vi "UTiLIA Main.vi"() -> ()   [LabVIEW 2022 SP3]
uses:
  <vilib>/Analysis/NI_AALPro.lvlib
  <vilib>/Analysis/5stat.llb/RMS (DBL).vi
  <vilib>/Utility/file.llb/Write To Spreadsheet File (DBL).vi
panel:
  in  "Sim?":bool
  out "Avg Temperature":dbl=296.9343435186893 format="%.1f"
  out "Nominal Resistance":dbl=0.0029999351419545705 format="%.2e"
  in  "Nom. Amplification":u16(ring)=3 items=["1", "10", "100", "1000", "10000"]
  out "Avg Quadrature Volt":dbl=-9.334672475592858e-06 format="%.5f"
  out "Long Avg Samp Volt":dbl=0.7499993324589096 format="%.6f"
  out "Avg Samp Volt":dbl=0.7499837854886428 format="%.6f"
  out "Measured Current":dbl=0.25000000000000006 format="%.0p"
  in  "Desired Current":dbl=0.25 format="%.0p"
  in  "Stop!":bool
  out "N=":i32=53
  in  "Calculate FFT?":bool=TRUE
  in  "Reset Avg?":bool
  out "Sampling Info":cluster{dbl[unit], i32}={71808.0, 16384} {"Hz" format="%.2f"}
  out "#S":i32=16384 caption="Samp/Chk"
  out "s/Samp":dbl[unit]=1.392602495543672e-05 format="%.0p"
  out "Fs":dbl[unit]=71808.0 caption="Samp Freq"
  out "Backlog":u32
  out "s/Chunk":dbl[unit]=0.2281639928698752 format="%.2f"
  out "s/Iter":dbl[unit]=0.13100000000849832 format="%.0p"
  in  "Reset Graph?":bool
  out "Resistance vs. Temp":cluster{dbl, dbl}[](graph)
  out "Error out":errorcluster
  in  "Save?":bool
  in  "Append?":bool
  in  "Data File":path=path "c:/users/flip/data/Test.txt"
  in  "Scale SV":dbl=1.0 min=0.0 max=2000.0 step=1.0 format="%.1p"
  out "Waveforms":dbl[][](graph)
  out "Mult Q":dbl[](array[numeric]) format="%.2f"
  out "Unit Reference":dbl[](array[numeric]) format="%.2f"
  out "Mult IP":dbl[](array[numeric]) format="%.2f"
  out "Applied Current":dbl[](array[numeric]) format="%.2f"
  out "Sample Voltage":dbl[](array[numeric]) format="%.2f"
  in  "Ref Freq":dbl[unit]=1122.0
  in  "Fs/Fref":u16=64 max=2000 step=20
  in  "Log S":i8=14 min=0 max=20 step=1
  out "Settle Time":dbl[unit]=0.025 format="%.1p"
  in  "Cutoff Freq":dbl[unit]=40.0 format="%.1f"
  in  "Filter Type":T1(ring)=enum."Inv Chebyshev"
  out "Avg Voltage vs. Time":T2(graph)={"Chunk Average"=0.7499837854886428, "Long-term Average"=0.7499993324589096, "Chunk Average"=-9.334672475592858e-06, 0.29693434351868925}
  out "FFT of Signal":cluster{"x":dbl, "df":dbl, dbl[]}[](graph)=[{"x"=0.0, "df"=4.3828125, array[8192 elements]}, {"x"=0.0, "df"=4.3828125, array[8192 elements]}, {"x"=0.0, "df"=4.3828125, array[8192 elements]}]
  out "Uncertainty Estimate":dbl[](graph)=[1.5546970266844262e-05]
  # "Save Data to File"
  # "Sampling Info"
  # "Averaged Values"
  # "Filter Info"
  # "Error Status"
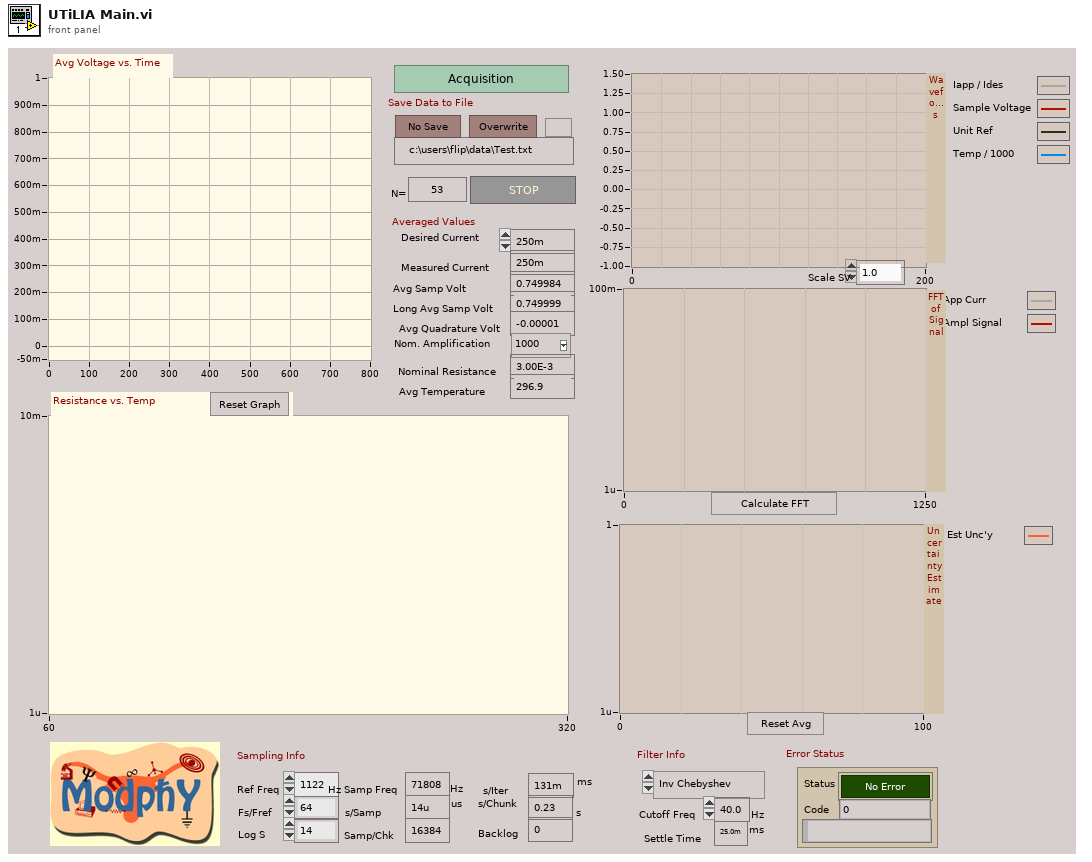
[diagram p1: front panel]
types:
  T1 = enum16{"None", "Butterworth", "Chebyshev", "Inv Chebyshev"}
  T2 = cluster{"Chunk Average":dbl, "Long-term Average":dbl, "Chunk Average":dbl, dbl}
  T3 = cluster{"Average mode":enum16{"No Averaging", "Linear", "Exponential"}, "# of averages":u32}
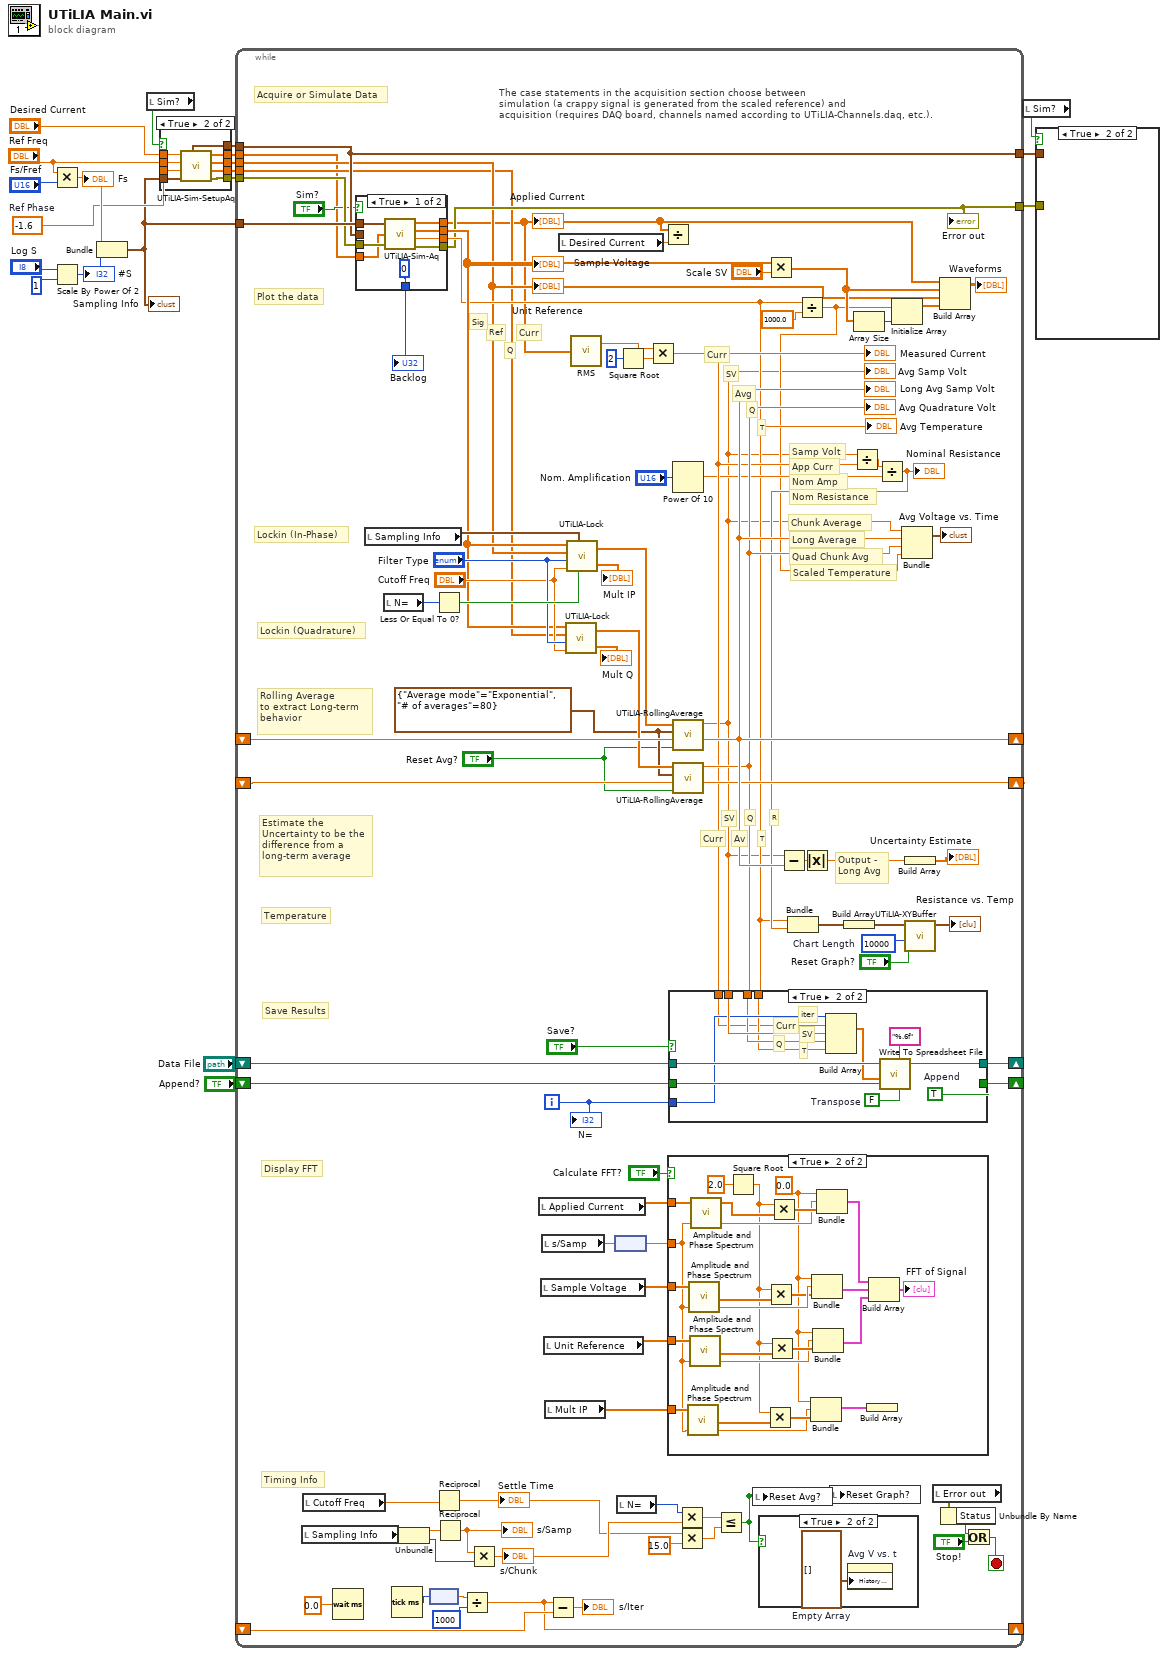
[diagram p0: block diagram]
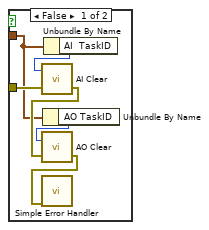
[diagram p2: hidden frame]
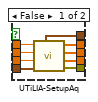
[diagram p3: hidden frame]
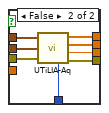
[diagram p4: hidden frame]
diagram:
  w6 = -1.6  # Ref Phase
  n1 = Multiply(x="Ref Freq", y="Fs/Fref") -> (x*y=w11:dbl[unit])
  "Fs" <- w11
  n2 = Scale By Power Of 2(n="Log S", x=1 ("n")) -> (x*2^n=w10:i32)
  "#S" <- w10
  n3 = Bundle(w11, w10) -> (w5:cluster{dbl[unit], i32})  [unwired: 1 in]
  "Sampling Info" <- w5
  n4 = local read "Sim?"() -> (w3:bool)
  n5 = case shown="True" w3 {
    tunnel: [w29 w38] -> w18
    tunnel: [w28 w37] -> w4
    tunnel: [w27 w36] -> w16
    tunnel: [w26 w35] -> w15
    tunnel: "Ref Freq" -> [w25 w34]
    tunnel: w5 -> [w24 w33]
    tunnel: "Desired Current" -> [w23 w32]
    tunnel: w6 -> [w22 w31]
    tunnel: [w21 w30] -> w2
    frame False {
      n6 = call "UTiLIA-SetupAq.vi"("Sampling Info"=w24, "Ref Phase"=w22, "Ref Frequency"=w25, "Ref Amplitude"=w23) -> ("Error out"=w29:errorcluster, "Unit Quadrature"=w26:dbl[], "Unit Reference"=w27:dbl[], "Scaled Reference"=w21:dbl[], "DAQ Configuration"=w28:cluster{"AO TaskID":u32, "AI  TaskID":u32})
    }
    frame True {
      n7 = call "UTiLIA-Sim-SetupAq.vi"("Sampling Info"=w33, "Ref Phase"=w31, "Ref Frequency"=w34, "Ref Amplitude"=w32) -> ("Error out"=w38:errorcluster, "Unit Quadrature"=w35:dbl[], "Unit Reference"=w36:dbl[], "Scaled Reference"=w30:dbl[], "DAQ Configuration"=w37:cluster{"AO TaskID":u32, "AI  TaskID":u32})
    }
  }
  n8 = while {
    shift-right: [w128] -> _
    shift-left: "Data File" -> [w127]
    shift-right: [w121] -> _
    shift-left: "Append?" -> [w126]
    shift-right: [w96] -> _
    shift-left: _ -> [w116]
    tunnel: w5 -> [w106]
    tunnel: w18 -> [w105]
    tunnel: [w55] -> w17
    tunnel: [w102] -> w9
    tunnel: w4 -> [w102]
    tunnel: w16 -> [w43]
    tunnel: w15 -> [w42]
    shift-right: [w59] -> _
    shift-left: _ -> [w87]
    shift-right: [w75] -> _
    shift-left: _ -> [w76]
    tunnel: w2 -> [w40]
    i -> [w107]
    stop <- w82 stop-if-true
    w74 = 10000  # Chart Length
    w77 = T3 {"Average mode"=enum."Exponential", "# of averages"=80} ("Rolling Avg Params")
    # "Plot the data"
    # "Acquire or Simulate Data"
    # "The case statements in the acquisition section choose between \nsimulation (a crappy signal is generated from the scaled reference) and\nacquisition (requires DAQ board, channels named according to UTiLIA-Channels.daq, etc.)."
    # "Curr"
    # "Nom Amp"
    # "Scaled Temperature"
    # "R"
    # "Nom Resistance"
    # "App Curr"
    # "Samp Volt"
    # "Quad Chunk Avg"
    # "Av"
    # "Curr"
    # "Curr"
    # "Q"
    # "Timing Info"
    # "Avg"
    # "T"
    # "SV"
    # "Q"
    # "Q"
    # "SV"
    # "Temperature"
    # "Display FFT"
    # "Save Results"
    # "T"
    # "Ref"
    # "Sig"
    # "Estimate the\nUncertainty to be the\ndifference from a \nlong-term average"
    # "Output -\nLong Avg"
    # "Long Average"
    # "Chunk Average"
    # "Rolling Average\nto extract Long-term \nbehavior"
    # "Lockin (Quadrature)"
    # "Lockin (In-Phase)"
    n9 = local read "Sampling Info"() -> (w125:cluster{dbl[unit], i32})
    n10 = local read "Cutoff Freq"() -> (w120:dbl[unit])
    n11 = Wait (ms)(milliseconds to wait=0.0) -> ()  [unwired: 1 out]
    n12 = case shown="True" "Sim?" {
      tunnel: w106 -> [w131 w144]
      tunnel: w105 -> [w136 w143]
      tunnel: [u32 0 ("Backlog") w142] -> w104
      tunnel: w102 -> [_ w141]
      tunnel: [w135 w140] -> w80
      tunnel: [w134 w139] -> w39
      tunnel: [w132 w138] -> w61
      tunnel: [w133 w137] -> w55
      tunnel: w40 -> [w130 _]
      frame True {
        n13 = call "UTiLIA-Sim-Aq.vi"("Sampling Info"=w131, "Scaled Reference"=w130, "Error in"=w136) -> ("Applied Current"=w134:dbl[], "Sample Voltage"=w135:dbl[], "Avg Temperature"=w132:dbl, "Error out"=w133:errorcluster)  [unwired: 1 in]
      }
      frame False {
        n14 = call "UTiLIA-Aq.vi"("Sampling Info"=w144, "DAQ Configuration"=w141, "Error in"=w143) -> ("Applied Current"=w139:dbl[], "Sample Voltage"=w140:dbl[], "Avg Temperature"=w138:dbl, "Error out"=w137:errorcluster, "Backlog"=w142:u32)
      }
    }
    "Backlog" <- w104
    "Sample Voltage" <- w80
    "Applied Current" <- w39
    "Avg Temperature" <- w61
    "Error out" <- w55
    n15 = local read "Sampling Info"() -> (w99:cluster{dbl[unit], i32})
    n16 = local read "N="() -> (w114:i32)
    n17 = Tick Count (ms)() -> (millisecond timer value=w88:u32)
    n18 = Unbundle(w125) -> (w123:dbl[unit], w124:i32)
    n19 = node(w88) -> (w54:dbl[unit])
    n20 = Less Or Equal To 0?(x=w114) -> (x <= 0?=w100:bool)
    n21 = Reciprocal(x=w120) -> (1/x=w110:dbl[unit])
    "Settle Time" <- w110
    n22 = Reciprocal(x=w123) -> (1/x=w122:dbl[unit])
    "s/Samp" <- w122
    n23 = Divide(x=w54, y=u32 1000) -> (x/y=w59:dbl[unit])
    n24 = Multiply(x=w122, y=w124) -> (x*y=w112:dbl[unit])
    "s/Chunk" <- w112
    n25 = local read "Applied Current"() -> (w90:dbl[])
    n26 = local read "Sample Voltage"() -> (w89:dbl[])
    n27 = local read "s/Samp"() -> (w49:dbl[unit])
    n28 = local read "Unit Reference"() -> (w91:dbl[])
    n29 = local read "Mult IP"() -> (w115:dbl[])
    n30 = Subtract(x=w59, y=w87) -> (x-y=→"s/Iter":dbl[unit])
    n31 = local read "Desired Current"() -> (w44:dbl)
    n32 = call "UTiLIA-Lock.vi"("Cutoff Freq"="Cutoff Freq", "Filter Type"="Filter Type", "Unit Reference"=w42, "Noisy Signal"=w80) -> ("Multiplied Signal"=→"Mult Q":dbl[], "Locked Signal"=w78:dbl[])  [unwired: 2 in]
    n33 = call "UTiLIA-Lock.vi"("Reset Filter?"=w100, "Sampling Info"=w99, "Cutoff Freq"="Cutoff Freq", "Filter Type"="Filter Type", "Unit Reference"=w43, "Noisy Signal"=w80) -> ("Multiplied Signal"=→"Mult IP":dbl[], "Locked Signal"=w97:dbl[])
    n34 = call-poly <vilib>:"RMS.vi"("X"=w39) -> ("rms value"=w67:dbl)  [unwired: 1 out]
    n35 = node(w49) -> (w50:dbl)
    n36 = local read "N="() -> (w113:i32)
    n37 = Square Root(x=2 ("y")) -> (sqrt(x)=w68:dbl)
    n38 = Multiply(x=w67, y=w68) -> (x*y=w66:dbl)
    "Measured Current" <- w66
    n39 = Divide(x=w39, y=w44) -> ()  [unwired: 1 out]
    n40 = case shown="True" "Calculate FFT?" {
      tunnel: w90 -> [_ w168]
      tunnel: w115 -> [_ w163]
      tunnel: w50 -> [_ w146]
      tunnel: w89 -> [_ w154]
      tunnel: w91 -> [_ w153]
      frame False {
      }
      frame True {
        w149 = 0.0 ("x")
        n41 = call <vilib>:"Amplitude and Phase Spectrum.vi"("dt"=w146, "Signal (V)"=w163) -> ("df"=w161:dbl, "Amp Spectrum Mag (Vrms)"=w164:dbl[])  [unwired: 1 in, 1 out]
        n42 = call <vilib>:"Amplitude and Phase Spectrum.vi"("dt"=w146, "Signal (V)"=w154) -> ("df"=w160:dbl, "Amp Spectrum Mag (Vrms)"=w159:dbl[])  [unwired: 1 in, 1 out]
        n43 = call <vilib>:"Amplitude and Phase Spectrum.vi"("dt"=w146, "Signal (V)"=w153) -> ("df"=w150:dbl, "Amp Spectrum Mag (Vrms)"=w151:dbl[])  [unwired: 1 in, 1 out]
        n44 = call <vilib>:"Amplitude and Phase Spectrum.vi"("dt"=w146, "Signal (V)"=w168) -> ("df"=w166:dbl, "Amp Spectrum Mag (Vrms)"=w169:dbl[])  [unwired: 1 in, 1 out]
        n45 = Square Root(x=2.0) -> (sqrt(x)=w148:dbl)
        n46 = Multiply(x=w148, y=w164) -> (x*y=w165:dbl[])
        n47 = Multiply(x=w148, y=w159) -> (x*y=w158:dbl[])
        n48 = Multiply(x=w148, y=w151) -> (x*y=w152:dbl[])
        n49 = Multiply(x=w148, y=w169) -> (x*y=w167:dbl[])
        n50 = Bundle("x"=w149, "df"=w161, w165) -> (w162:cluster{"x":dbl, "df":dbl, dbl[]})  [unwired: 1 in]
        n51 = Bundle("x"=w149, "df"=w160, w158) -> (w155:cluster{"x":dbl, "df":dbl, dbl[]})  [unwired: 1 in]
        n52 = Bundle("x"=w149, "df"=w150, w152) -> (w147:cluster{"x":dbl, "df":dbl, dbl[]})  [unwired: 1 in]
        n53 = Bundle("x"=w149, "df"=w166, w167) -> (w156:cluster{"x":dbl, "df":dbl, dbl[]})  [unwired: 1 in]
        n54 = Build Array(w162) -> ()  [unwired: 1 out]
        n55 = Build Array(w156, w155, w147) -> (→"FFT of Signal":cluster{"x":dbl, "df":dbl, dbl[]}[])
      }
    }
    n56 = Power Of 10(x="Nom. Amplification") -> (10^x=w63:dbl)
    n57 = call "UTiLIA-RollingAverage.vi"("Restart Avg"="Reset Avg?", "Current Average"=w116, "Rolling Avg Parameters"=w77, "Signal to Average"=w97) -> ("Long-term Average"=w96:dbl, "Chunk Average"=w48:dbl)  [unwired: 3 out]
    "Avg Samp Volt" <- w48
    "Long Avg Samp Volt" <- w96
    n58 = call "UTiLIA-RollingAverage.vi"("Restart Avg"="Reset Avg?", "Current Average"=w76, "Rolling Avg Parameters"=w77, "Signal to Average"=w78) -> ("Long-term Average"=w75:dbl, "Chunk Average"=w71:dbl)  [unwired: 3 out]
    "Avg Quadrature Volt" <- w71
    n59 = case shown="True" "Save?" {
      tunnel: [w172 w183] -> w128
      tunnel: w127 -> [w172 w182]
      tunnel: w126 -> [w171 w181]
      tunnel: [w171 w179] -> w121
      tunnel: w48 -> [_ w178]
      tunnel: w61 -> [_ w174]
      tunnel: w107 -> [_ w176]
      tunnel: w71 -> [_ w175]
      tunnel: w66 -> [_ w173]
      frame False {
      }
      frame True {
        w179 = TRUE  # Append
        w180 = FALSE  # Transpose
        # "Curr"
        # "Q"
        # "SV"
        # "T"
        # "iter"
        n60 = Build Array(w176, w173, w178, w175, w174) -> (w177:dbl[])
        n61 = call-poly <vilib>:"Write To Spreadsheet File.vi"("transpose? (no:F)"=w180, "format (%.3f)"="%.6f", "append to file? (new file:F)"=w181, "1D data"=w177, "file path (dialog if empty)"=w182) -> ("new file path (Not A Path if cancelled)"=w183:path)  [unwired: 3 in]
      }
    }
    n62 = Multiply(x=w113, y=w112) -> (x*y=w111:dbl[unit])
    n63 = Multiply(x=w110, y=15.0 ("x")) -> (x*y=w109:dbl[unit])
    n64 = Less Or Equal?(x=w111, y=w109) -> (x <= y?=w45:bool)
    n65 = local write "Reset Avg?"(w45) -> ()
    n66 = case shown="True" w45 {
      frame False {
      }
      frame True {
        w145 = cluster{dbl, dbl, dbl, dbl}[] []  # Empty Array
        n67 = property on="Avg V vs. t" class="WFChart (strict)"("History Data"=w145) -> ()  [unwired: 2 in, 2 out]
      }
    }
    n68 = Multiply(x=w80, y="Scale SV") -> (x*y=w81:dbl[])
    n69 = Subtract(x=w48, y=w96) -> (x-y=w118:dbl)
    n70 = Divide(x=w61, y=1000.0) -> (x/y=w52:dbl)
    n71 = Absolute Value(x=w118) -> (abs(x)=w117:dbl)
    n72 = local write "Reset Graph?"(w45) -> ()
    n73 = Divide(x=w48, y=w66) -> (x/y=w65:dbl)
    n74 = Array Size(array=w81) -> (size(s)=w98:i32)
    n75 = Divide(x=w65, y=w63) -> (x/y=w62:dbl)
    "Nominal Resistance" <- w62
    n76 = Bundle("Avg Temperature"=w61, w62) -> (w72:cluster{"Avg Temperature":dbl, dbl})  [unwired: 1 in]
    n77 = Build Array(w72) -> (w73:cluster{"Avg Temperature":dbl, dbl}[])
    n78 = Initialize Array(w52, w98) -> (w95:dbl[])
    n79 = Bundle("Chunk Average"=w48, "Long-term Average"=w96, "Chunk Average"=w71, w52) -> (→"Avg Voltage vs. Time":T2)  [unwired: 1 in]
    n80 = Build Array(w117) -> (→"Uncertainty Estimate":dbl[])
    n81 = call "UTiLIA-XYBuffer.vi"("clear first (no:F)"="Reset Graph?", "chart length (points)"=w74, "new points"=w73) -> ("XY chart data"=→"Resistance vs. Temp":cluster{"x":dbl, "y":dbl}[])  [unwired: 8 in]
    n82 = local read "Error out"() -> (w85:errorcluster)
    n83 = Build Array(w39, w81, w43, w95) -> (→"Waveforms":dbl[][])
    n84 = Unbundle By Name(w85) -> ("Status"=w84:bool)
    n85 = Or(x=w84, y="Stop!") -> (x .or. y?=w82:bool)
    "N=" <- w107
    "Unit Reference" <- w43
  }
  n86 = local read "Sim?"() -> (w1:bool)
  n87 = case shown="True" w1 {
    tunnel: w17 -> [w190 _]
    tunnel: w9 -> [w187 _]
    frame False {
      n88 = Unbundle By Name(w187) -> ("AO TaskID"=w185:u32)
      n89 = Unbundle By Name(w187) -> ("AI  TaskID"=w186:u32)
      n90 = call "AI Clear.vi"("error in (no error)"=w190, "taskID in"=w186) -> ("error out"=w189:errorcluster)  [unwired: 4 in, 1 out]
      n91 = call "AO Clear.vi"("error in (no error)"=w189, "taskID in"=w185) -> ("error out"=w188:errorcluster)  [unwired: 4 in, 1 out]
      n92 = call <vilib>:"Simple Error Handler.vi"("error in (no error)"=w188) -> ()  [unwired: 4 in, 5 out]
    }
    frame True {
    }
  }
